vi "Is Triggered.vi"(8 "error in (no error)":errorcluster, 11 "DAQmx Recorder in":refnum<class "DAQmx Recorder.lvclass">) -> (0 "error out":errorcluster, 2 "Triggered":bool, 3 "DAQmx Recorder out":refnum<class "DAQmx Recorder.lvclass">)   [LabVIEW 2015, in "DAQmx Recorder.lvclass"]
uses:
  DAQmx Recorder.lvclass
  DAQmx Recorder.lvclass/DAQmx Recorder.ctl
  NHMFL_Core/Libraries/NI-DAQ/DAQmx Digitizer/DAQmx Digitizer.lvclass
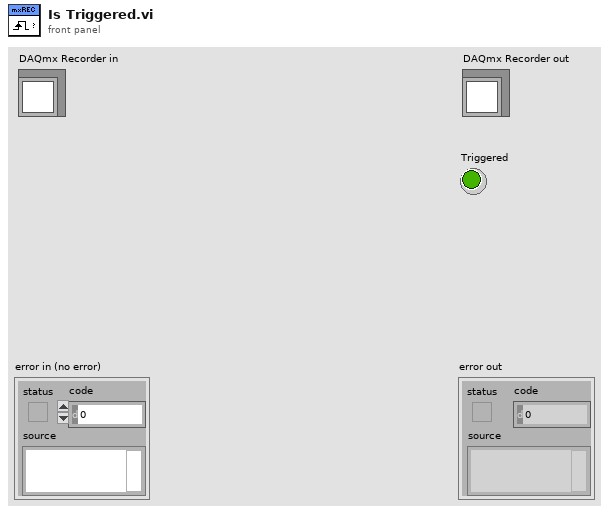
[diagram p1: front panel]
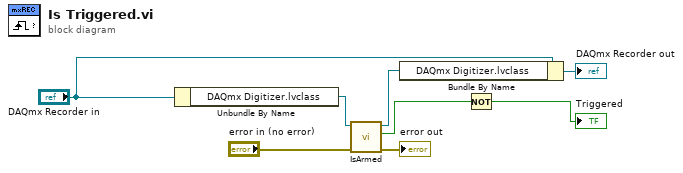
[diagram p0: block diagram]
diagram:
  n1 = Unbundle By Name("DAQmx Recorder in") -> ("DAQmx Digitizer.lvclass"=w7:refnum<class "DAQmx Digitizer.lvclass">)
  n2 = call-dynamic "IsArmed.vi"("error in (no error)"="error in (no error)", "DAQmx Digitizer in"=w7) -> ("error out"=→"error out":errorcluster, "Armed"=w2:bool, "DAQmx Digitizer out"=w3:refnum<class "DAQmx Digitizer.lvclass">)  [unwired: 5 in, 2 out]
  n3 = Bundle By Name(cluster="DAQmx Recorder in", "DAQmx Digitizer.lvclass"=w3) -> (→"DAQmx Recorder out":refnum<class "DAQmx Recorder.lvclass">)
  n4 = Not(x=w2) -> (.not. x?=→"Triggered":bool)
